vi "Initialize.vi"(9 "Column":i32, 10 "Row":i32, 11 "Starter in":refnum<class "Starter.lvclass">) -> (3 "Fortress out":refnum<class "Fortress.lvclass">)   [LabVIEW 2015, in "Starter.lvclass"]
uses:
  Starter.lvclass
  Fortress/Fortress.lvclass
  Common/Position.ctl
  Starter.lvclass/Starter.ctl
  Common/Common.lvlib
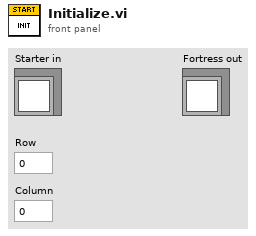
[diagram p1: front panel]
types:
  T1 = typedef "Common.lvlib/Position.ctl" = cluster{"Column":i32, "Row":i32}
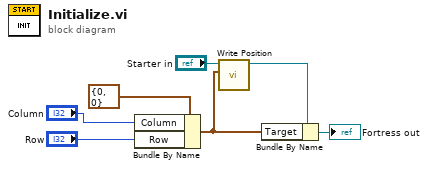
[diagram p0: block diagram]
diagram:
  n1 = Bundle By Name(cluster=T1 {"Column"=0, "Row"=0} ("Center"), "Column"="Column", "Row"="Row") -> (w1:T1)
  n2 = call-dynamic "Write Position.vi"("Position"=w1, "Fortress in"="Starter in") -> ("Fortress out"=w2:refnum<class "Starter.lvclass">)  [unwired: 8 in, 1 out]
  n3 = Bundle By Name(cluster=w2, "Target"=w1) -> (→"Fortress out":refnum<class "Starter.lvclass">)
